vi "Global Megger.vi"() -> ()   [LabVIEW 2014]
panel:
  in  "VISA resource name out":refnum<visa-resource-name>
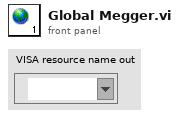
[diagram p1: front panel]
diagram:
